vi "Secret.vi"() -> ()   [LabVIEW 2016]
panel:
  in  "Number":dbl
  in  "Suprise":bool
  in  "Secret":bool
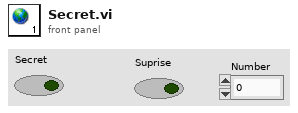
[diagram p1: front panel]
diagram:
